vi "PH_Beamline_Chief.constructor.vi"(0 "name":string, 2 "data in":string, 5 "error in":errorcluster) -> (14 "i ref out":refnum<vi>, 16 "data out":string, 19 "error out":errorcluster)   [LabVIEW 2014, in "PH_Beamline_Chief.lvlib"]
doc: "This class is forseen to inspect the PHELIX beamline and to select the mode. Additional several settings can be chosen.\n\nThis class is part of the PHELIX user layer.\n\nauthor: Stefan Götte, GSI\n\nLicense Agreement for this software:\n\nCopyright (C)\nGesellschaft für Schwerionenforschung, GSI\nPlanckstr. 1\n64291 Darmstadt\nGermany\n\nContact: D.Beck@gsi.de \n\nThis program is free software; you can redistribute it and/or modify it under the terms of the \nGNU General Public License as published by the Free Software Foundation; either version 2 of \nthe license, or (at your option) any later version.\n\nThis program is distributed in the hope that it will be useful, but WITHOUT ANY WARRANTY; \nwithout even the implied warranty of MERCHANTABILITY or FITNESS FOR A PARTICULAR PURPOSE. See the GNU General License for more details (http://www.gnu.org).\n\nGesellschaft für Schwerionenforschung, GSI\nPlanckstr. 1, 64291 Darmstadt, Germany\nFor all questions and ideas contact: M.Richter@gsi.de, H.Brand@gsi.de or D.Beck@gsi.de.\nLast update: 16-JUN-2004"
uses:
  PH_Beamline_Chief.lvlib
  CSCore/CSSystem/CSSystemLib/CSSystemLib.lvlib
  PH_Beamline/PH_Beamline.lvlib
  CSCore/CSObj/CSObj.lvlib
  PH_Class/PH_Class.lvlib
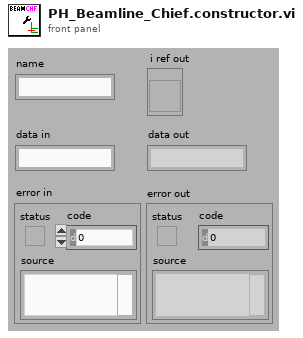
[diagram p1: front panel]
types:
  T1 = enum16{"SetAttribute", "GetAttribute", "CreateAttribute", "DestroyAttribute", "DestroyAllAtributes"}
  T2 = typedef "PH_Beamline_Chief.lvlib/PH_Beamline_Chief.i attribute.ctl" = cluster{"BL Service IDs":cluster{"YLF_BL_Status":i32, "fs_BL_Status":i32, "fs_YLF_BL_Status":i32, "ns_BL_Status":i32, "PA_Input_BL_Status":i32, "PA_UnDelay_BL_Status":i32, "PA_Delay_BL_Status":i32, "PA_BL_Status":i32, "PA_Bypass_BL_Status":i32, "PA_Exit_BL_Status":i32, "PA_LL_BL_Status":i32, "LL_BL_Status":i32, "PA_MA_BL_Status":i32, "MA_Exit_BL_Status":i32, "MA_Z6_BL_Status":i32, "Z6_BL_Status":i32, "MA_LB_BL_Status":i32, "LB_TB2_BL_Status":i32, "PA_before_Bypass_BL_Status":i32, "LB_TB3_BL_Status":i32}, "R2S Service ID":i32, "Settings":cluster{"Wanted":T3, "GUI Ref":refnum<vi>, "Service ID":i32}}
  T3 = typedef "PH_Beamline_Chief.lvlib/PH_Beamline_Chief.Settings.ctl" = cluster{"PA Doublepass Mode":bool, "Compressor Vaccuum LB not relevant":bool, "Windowshutter TB2 not relevant":bool, "Windowshutter TB3 not relevant":bool}
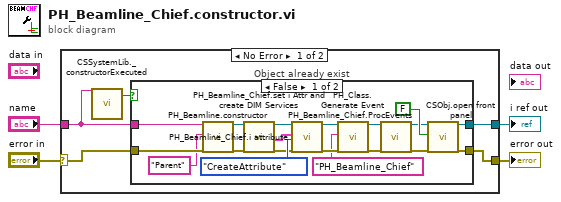
[diagram p0: block diagram]
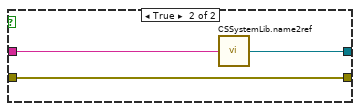
[diagram p2: hidden frame]
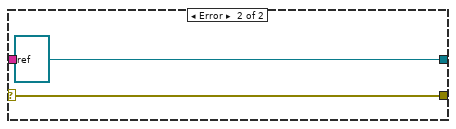
[diagram p3: hidden frame]
diagram:
  n1 = case shown="No Error" "error in" {
    selector: "error in" -> [w5 w33]
    tunnel: "name" -> [w6 _]
    tunnel: [w8 w33] -> w3
    tunnel: [w7 refnum<vi> refnum ("i ref out")] -> w2
    frame No Error {
      n2 = call "CSSystemLib._constructorExecuted.vi"("name"=w6) -> ("constructor executed?"=w9:bool)  [unwired: 18 in]
      n3 = case "Object already exist" shown="False" w9 {
        tunnel: w6 -> [w27 w31]
        tunnel: [w19 w30] -> w8
        tunnel: w5 -> [w21 w30]
        tunnel: [w20 w29] -> w7
        frame False {
          n4 = call "PH_Beamline.constructor.vi"("name"=w27, "data in"="Parent", "error in"=w21) -> ("i ref out"=w22:refnum<vi>, "error out"=w23:errorcluster)  [unwired: 14 in, 1 out]
          n5 = call "PH_Beamline_Chief.set i Attr and create DIM Services.vi"("Refnum in"=w22, "error in"=w23) -> ("i ref out"=w26:refnum<vi>, "i Attr"=w24:T2, "error out"=w25:errorcluster)  [unwired: 15 in]
          n6 = call "PH_Beamline_Chief.i attribute.vi"("VI Refnum"=w26, "CLASS.i attribute"=w24, "Action"=T1."CreateAttribute", "error in (no error)"=w25) -> ("VI Refnum out"=w17:refnum<vi>, "error out"=w16:errorcluster)  [unwired: 13 in, 1 out]
          n7 = call "PH_Class.Generate Event.vi"("i ref in"=w17, "Class"="PH_Beamline_Chief", "error in (no error)"=w16) -> ("i ref out"=w12:refnum<vi>, "error out"=w15:errorcluster)  [unwired: 15 in]
          n8 = call "PH_Beamline_Chief.ProcEvents.vi"("i ref in"=w12, "error in (no error)"=w15) -> ("i ref out"=w11:refnum<vi>, "error out"=w13:errorcluster)  [unwired: 16 in]
          n9 = call "CSObj.open front panel.vi"("i ref in"=w11, "frontPanelOpen"=FALSE, "error in (no error)"=w13) -> ("i ref out"=w20:refnum<vi>, "error out"=w19:errorcluster)  [unwired: 15 in]
        }
        frame True {
          n10 = call "CSSystemLib.name2ref.vi"("name"=w31) -> ("obj refnum"=w29:refnum<vi>)
        }
      }
    }
    frame Error {
    }
  }
  "i ref out" <- w2
  "error out" <- w3
